vi "Tetris_on_FPGA.vi"   [LabVIEW 2018]
panel:
  # "Tetris on FPGA\nCreated by Pascal Heinen\npascal@vi-tech.nl\nVI Technologies"
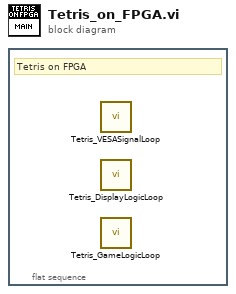
[diagram p0: block diagram]
diagram:
  n1 = flat-sequence {
    frame #0 {
      # "Tetris on FPGA"
      n2 = call "Tetris_VESASignalLoop.vi"() -> ()  [unwired: 12 in]
      n3 = call "Tetris_DisplayLogicLoop.vi"() -> ()  [unwired: 12 in]
      n4 = call "Tetris_GameLogicLoop.vi"() -> ()  [unwired: 20 in]
    }
  }
